vi "TranslateVI.vi"(8 "error in (no error)":errorcluster, 9 "Target Language":string, 10 "Dictionary":string[][](array[string]), 11 "VI in":refnum<vi>) -> (0 "error out":errorcluster)   [LabVIEW 2017, in "JKI Simple Localization.lvlib"]
uses:
  API/JKI Simple Localization.lvlib
  <vilib>/Utility/traverseref.llb/TRef TravTarget.ctl
  <vilib>/Utility/traverseref.llb/VI Scripting - Traverse.lvlib
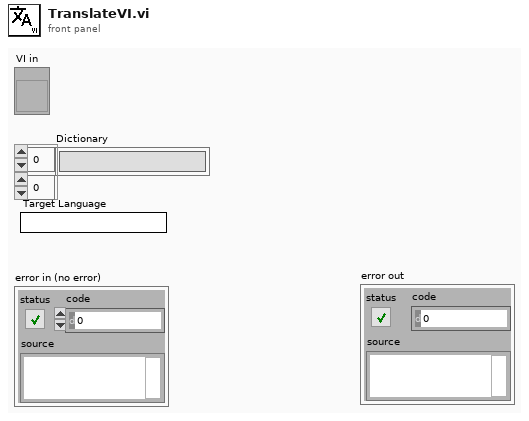
[diagram p1: front panel]
types:
  T1 = typedef "TRef TravTarget.ctl" = enum16{"FP", "BD", "Other"}
  T2 = typedef "JKI Simple Localization.lvlib/Font Info.ctl" = cluster{"Custom Font Color":bool, "Font Color":u32, "Custom Font Name":bool, "Font Name":string}
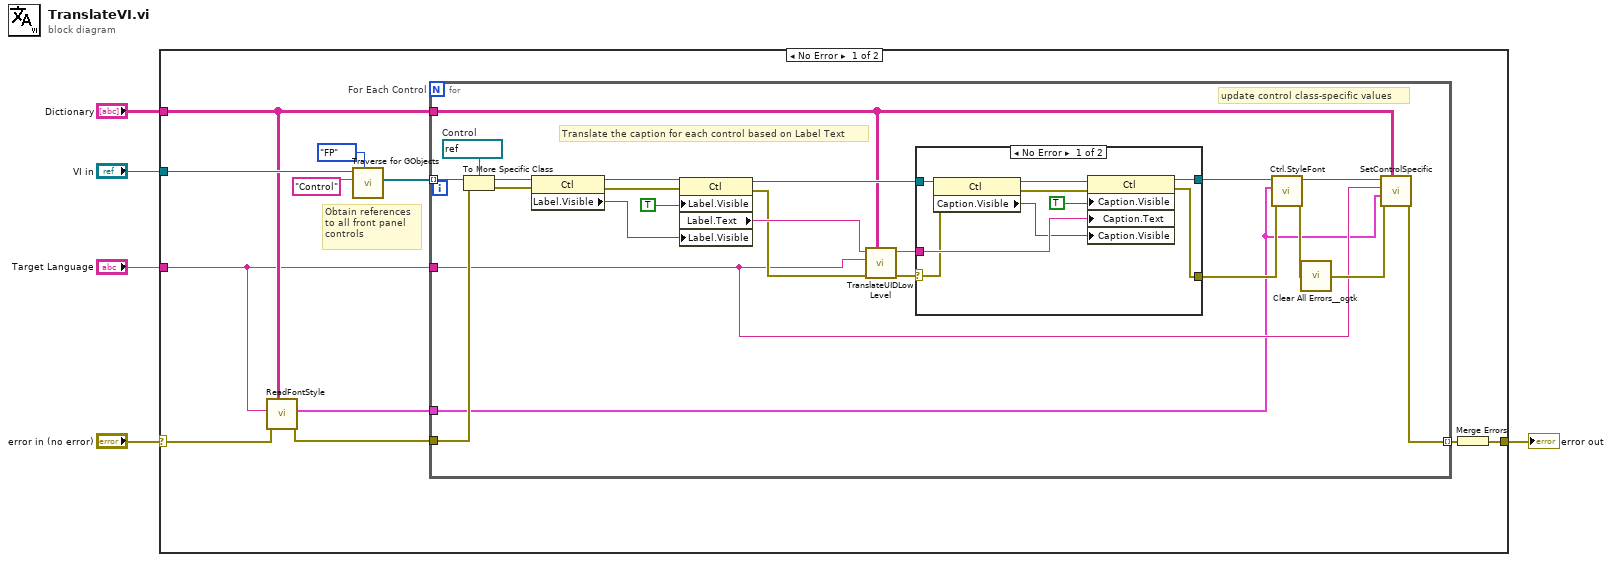
[diagram p0: block diagram]
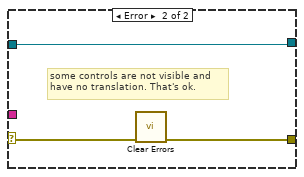
[diagram p2: hidden frame]
diagram:
  n1 = case shown="No Error" "error in (no error)" {
    selector: "error in (no error)" -> [w7 w52]
    tunnel: "VI in" -> [w14 _]
    tunnel: [w11 w52] -> w4
    tunnel: "Dictionary" -> [w9 _]
    tunnel: "Target Language" -> [w8 _]
    frame No Error {
      # "Obtain references to all front panel controls"
      n2 = call "ReadFontStyle.vi"("Dictionary"=w9, "error in (no error)"=w7, "Target Language"=w8) -> ("error out"=w10:errorcluster, "Font Info"=w6:T2)  [unwired: 7 in]
      n3 = call <vilib>:"Traverse for GObjects.vi"("Traverse Target"=TRef_TravTarget."FP", "Class Name"="Control", "VI Refnum"=w14) -> ("References"=w15:refnum<vi>[])  [unwired: 5 in, 3 out]
      n4 = for "For Each Control" {
        tunnel: w15 -> [w39] mode=indexing
        tunnel: w10 -> [w37]
        tunnel: w9 -> [w25]
        tunnel: w8 -> [w22]
        tunnel: [w24] -> w16 mode=indexing
        tunnel: w6 -> [w17]
        w38 = refnum<vi> refnum  # Control
        # "update control class-specific values"
        # "Translate the caption for each control based on Label Text"
        n5 = To More Specific Class(target class=w38, reference=w39, error in=w37) -> (specific class reference=w35:refnum<vi>, error out=w29:errorcluster)
        n6 = property class="Ctl"(reference=w35, error in=w29) -> (reference out=w34:refnum<vi>, error out=w28:errorcluster, "Label.Visible"=w33:bool)
        n7 = property class="Ctl"(reference=w34, error in=w28, "Label.Visible"=TRUE, "Label.Visible"=w33) -> (reference out=w30:refnum<vi>, error out=w27:errorcluster, "Label.Text"=w36:string)
        n8 = call "TranslateUIDLowLevel.vi"("Dictionary"=w25, "error in (no error)"=w27, "Target Language"=w22, "UID"=w36) -> ("error out"=w26:errorcluster, "Translated Word"=w31:string)  [unwired: 6 in]
        n9 = case shown="No Error" w26 {
          selector: w26 -> [w41 w51]
          tunnel: w31 -> [w47 _]
          tunnel: w30 -> [w46 w49]
          tunnel: [w42 w50] -> w19
          tunnel: [w40 w49] -> w21
          frame No Error {
            n10 = property class="Ctl"(reference=w46, error in=w41) -> (reference out=w45:refnum<vi>, error out=w43:errorcluster, "Caption.Visible"=w44:bool)
            n11 = property class="Ctl"(reference=w45, error in=w43, "Caption.Visible"=TRUE, "Caption.Text"=w47, "Caption.Visible"=w44) -> (reference out=w40:refnum<vi>, error out=w42:errorcluster)
          }
          frame Error {
            # "some controls are not visible and \nhave no translation. That's ok."
            n12 = call <vilib>:"Clear Errors.vi"("error in (no error)"=w51) -> ("error out"=w50:errorcluster)  [unwired: 5 in, 1 out]
          }
        }
        n13 = call "Ctrl.StyleFont.vi"("error in (no error)"=w19, "Font Info"=w17, "Ctl Ref in"=w21) -> ("error out"=w18:errorcluster, "Ctl Ref out"=w20:refnum<vi>)  [unwired: 7 in]
        n14 = call <userlib>:"Clear All Errors__ogtk.vi"("Error In"=w18) -> ("Error Out"=w23:errorcluster)  [unwired: 3 in]
        n15 = call "SetControlSpecific.vi"("Dictionary"=w25, "error in (no error)"=w23, "Font Info"=w17, "Target Language"=w22, "Control Reference"=w20) -> ("error out"=w24:errorcluster)  [unwired: 5 in, 1 out]
      }
      n16 = Merge Errors(w16) -> (w11:errorcluster)
    }
    frame Error {
    }
  }
  "error out" <- w4
